vi "Analog_Selector.vi"(3 "Test Name":string(combo)="Door Lock", 4 "Lane Number":string(combo)="Lane 1", 5 "Analog Data In":dbl[](array[numeric])) -> (0 "Volt 2":dbl, 1 "Volt 1":dbl, 2 "Force":dbl)   [LabVIEW 2017]
panel:
  out "V2 index":i32
  out "V1 index":i32
  out "Force index":i32
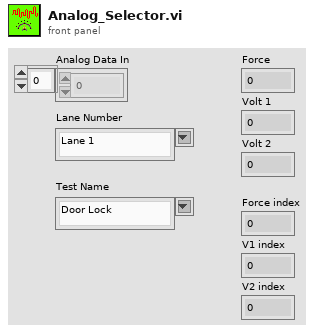
[diagram p1: front panel]
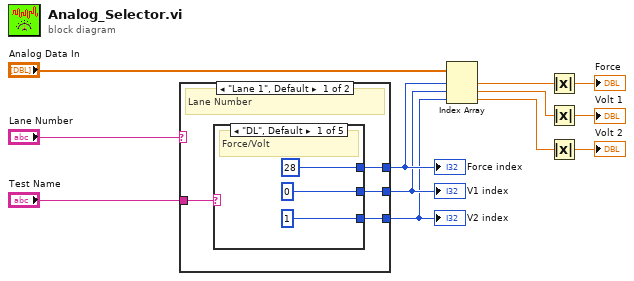
[diagram p0: block diagram]
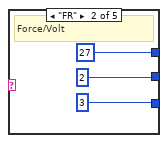
[diagram p2: hidden frame]
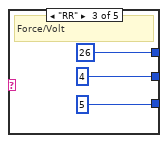
[diagram p3: hidden frame]
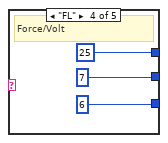
[diagram p4: hidden frame]
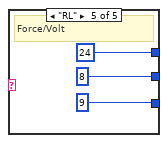
[diagram p5: hidden frame]
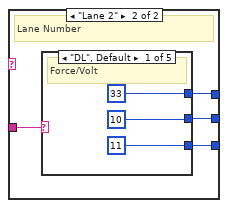
[diagram p6: hidden frame]
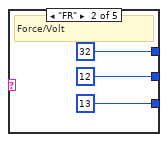
[diagram p7: hidden frame]
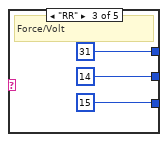
[diagram p8: hidden frame]
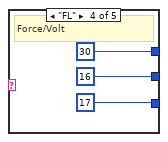
[diagram p9: hidden frame]
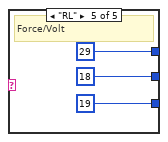
[diagram p10: hidden frame]
diagram:
  n1 = case shown="\"Lane 1\", Default" "Lane Number" {
    tunnel: "Test Name" -> [w13 w32]
    tunnel: [w16 w35] -> w9
    tunnel: [w15 w34] -> w4
    tunnel: [w14 w33] -> w3
    frame "Lane 1", Default {
      # "Lane Number"
      n2 = case shown="\"DL\", Default" w13 {
        tunnel: [28 ("index") 27 ("index") 26 ("index") 25 ("index") 24 ("index")] -> w16
        tunnel: [0 ("index") 2 ("index") 4 ("index") 7 ("index") 8 ("index")] -> w15
        tunnel: [1 ("index") 3 ("index") 5 ("index") 6 ("index") 9 ("index")] -> w14
        frame "DL", Default {
          # "Force/Volt"
        }
        frame "FR" {
          # "Force/Volt"
        }
        frame "RR" {
          # "Force/Volt"
        }
        frame "FL" {
          # "Force/Volt"
        }
        frame "RL" {
          # "Force/Volt"
        }
      }
    }
    frame "Lane 2" {
      # "Lane Number"
      n3 = case shown="\"DL\", Default" w32 {
        tunnel: [33 ("index") 32 ("index") 31 ("index") 30 ("index") 29 ("index")] -> w35
        tunnel: [10 ("index") 12 ("index") 14 ("index") 16 ("index") 18 ("index")] -> w34
        tunnel: [11 ("index") 13 ("index") 15 ("index") 17 ("index") 19 ("index")] -> w33
        frame "DL", Default {
          # "Force/Volt"
        }
        frame "FR" {
          # "Force/Volt"
        }
        frame "RR" {
          # "Force/Volt"
        }
        frame "FL" {
          # "Force/Volt"
        }
        frame "RL" {
          # "Force/Volt"
        }
      }
    }
  }
  "Force index" <- w9
  "V1 index" <- w4
  "V2 index" <- w3
  n4 = Index Array(array="Analog Data In", index #1=w9, index #2=w4, index #3=w3) -> (element #1=w11:dbl, element #2=w10:dbl, element #3=w5:dbl)
  n5 = Absolute Value(x=w11) -> (abs(x)=→"Force":dbl)
  n6 = Absolute Value(x=w10) -> (abs(x)=→"Volt 1":dbl)
  n7 = Absolute Value(x=w5) -> (abs(x)=→"Volt 2":dbl)
